vi "WPI_CompressorStop.vi"(8 "error in (no error)":errorcluster, 11 "CompressorDevRef":T1) -> (0 "error out":errorcluster, 3 "CompressorDevRef":T1)   [LabVIEW 2017]
doc: "Stops the compressor that you specify.\n\nThis software is licensed. Open the labview\\readme\\WPI Robotics Library Open Source License.txt file for more information."
uses:
  <vilib>/Rock Robotics/WPI/Compressor/WPI_CompressorDevRef.ctl
  <vilib>/Rock Robotics/WPI/CAN/PCM/WPI_CAN_PCMGlobalOps.ctl
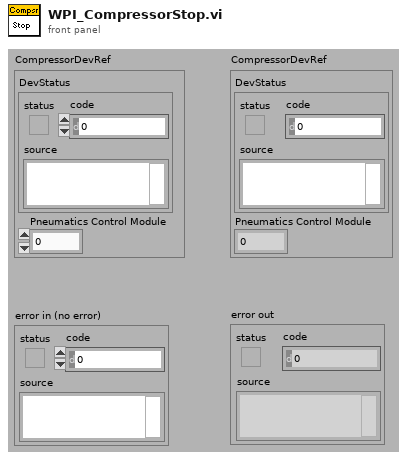
[diagram p1: front panel]
types:
  T1 = typedef "WPI_CompressorDevRef.ctl" = cluster{"DevStatus":errorcluster, "Pneumatics Control Module":u8}
  T2 = typedef "WPI_CAN_PCMGlobalOps.ctl" = enum16{"Read For Send", "Write After Receive", "Set Solenoids", "Set Closed Loop", "Clear Sticky Faults", "Get All", "Write Error", "Write After Receive Blacklist", "Set Control Frame Rate"}
  T3 = cluster{"Solenoid Status":bool[], "Battery Voltage":dbl, "Solenoid Voltage":dbl, "Compressor Current":dbl, "CompressorEnabled":bool, "StickySolenoidFault":bool, "StickyCompressorFault":bool, "SolenoidFault":bool, "CompressorFault":bool, "HardwareFault":bool, "ClosedLoopStatus":bool, "PressureStatus":bool, "Module Enabled":bool, "ClosedLoopSuggestedOutput":bool, "CAN Error":errorcluster, "Sticky Solenoid Faults":bool[]}
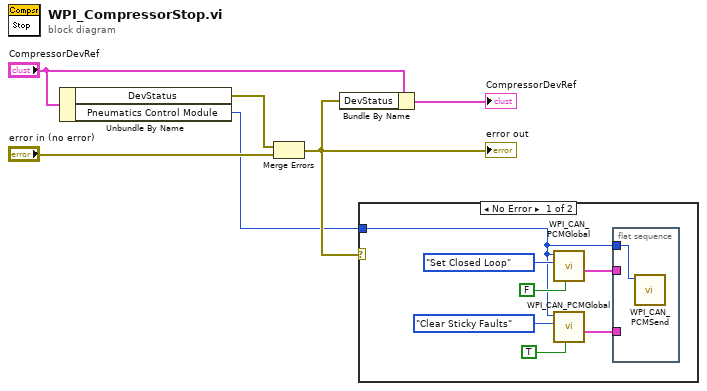
[diagram p0: block diagram]
diagram:
  n1 = Unbundle By Name("CompressorDevRef") -> ("DevStatus"=w3:errorcluster, "Pneumatics Control Module"=w1:u8)
  n2 = Merge Errors(w3, "error in (no error)") -> (w5:errorcluster)
  "error out" <- w5
  n3 = Bundle By Name(cluster="CompressorDevRef", "DevStatus"=w5) -> (→"CompressorDevRef":T1)
  n4 = case shown="No Error" w5 {
    tunnel: w1 -> [w9 _]
    frame No Error {
      n5 = call <vilib>:"WPI_CAN_PCMGlobal.vi"("Set Value"=FALSE, "Operation"=WPI_CAN_PCMGlobalOps."Set Closed Loop", "Pneumatics Control Module (0)"=w9) -> ("Get All"=w7:T3)  [unwired: 6 in, 2 out]
      n6 = call <vilib>:"WPI_CAN_PCMGlobal.vi"("Set Value"=TRUE, "Operation"=WPI_CAN_PCMGlobalOps."Clear Sticky Faults", "Pneumatics Control Module (0)"=w9) -> ("Get All"=w8:T3)  [unwired: 6 in, 2 out]
      n7 = flat-sequence {
        tunnel: w9 -> [w14]
        tunnel: w8 -> [_]
        tunnel: w7 -> [_]
        frame #0 {
          n8 = call <vilib>:"WPI_CAN_PCMSend.vi"("Pneumatics Control Module (0)"=w14) -> ()  [unwired: 10 in, 1 out]
        }
      }
    }
    frame Error {
    }
  }
